vi "VIWeverson.vi"   [LabVIEW 2024]
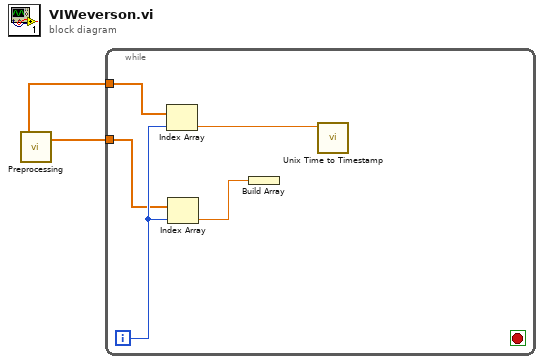
[diagram p0: block diagram]
diagram:
  n1 = call "Preprocessing.vi"() -> ("Potência Ativa A"=w1:dbl[], "timestamp"=w2:dbl[])  [unwired: 2 out]
  n2 = while {
    tunnel: w2 -> [w6]
    tunnel: w1 -> [w5]
    i -> [w7]
    stop <- _ stop-if-true
    n3 = Index Array(array=w6, index=w7) -> (element=w4:dbl)
    n4 = Index Array(array=w5, index=w7) -> (element=w3:dbl)
    n5 = Build Array(w3) -> ()  [unwired: 1 out]
    n6 = call <vilib>:"Unix Time to Timestamp.vi"("Unix Time (s)"=w4) -> ()  [unwired: 9 in, 2 out]
  }
